vi "output_byte.vi"() -> ()   [LabVIEW 2015]
uses:
  states.ctl
panel:
  out "Current State":T1
  out "Motors output":bool[](array[boolean])
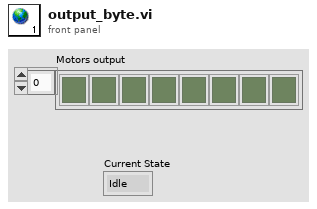
[diagram p1: front panel]
types:
  T1 = typedef "states.ctl" = enum16{"Idle", "Pause", "Next Contour", "Aligning", "Lowering Pen", "Drawing", "Next Point", "Lifting Pen", "Stop", "Put Away"}
diagram:
